vi "runTestScenario.vi"(8 "error in (no error)":errorcluster, 11 "Constant Analog Output Voltage Test  in":refnum<class "Modulated Analog Output Voltage Test.lvclass">) -> (0 "error out":errorcluster, 1 "Result":T1, 2 "TestExecution":T2, 3 "Constant Analog Output Voltage Test  out":refnum<class "Modulated Analog Output Voltage Test.lvclass">)   [LabVIEW 2015, in "Modulated Analog Output Voltage Test.lvclass"]
uses:
  Modulated Analog Output Voltage Test.lvclass
  Typedefs/TestExecution.ctl
  Typedefs/PassFailTest.ctl
  Modulated Analog Output Voltage Test.lvclass/Modulated Analog Output Voltage Test.ctl
  Typedefs/WriteDataFileInput.ctl
  Typedefs/TestScenarioTypes.ctl
  Typedefs/WriteLogMessageInput.ctl
  <vilib>/express/express arith-compare/Formula/XNode/ExpressFormulaBlockNode.xnode
  Model/TestLog/ITestLog/ITestLog.lvclass
  Model/ConverterStrategy/IConverterStrategy/IConverterStrategy.lvclass
  Model/ConfigureILCStrategy/IConfigureILCStrategy/IConfigureILCStrategy.lvclass
  Typedefs/ILCBTTypedefs.lvlib
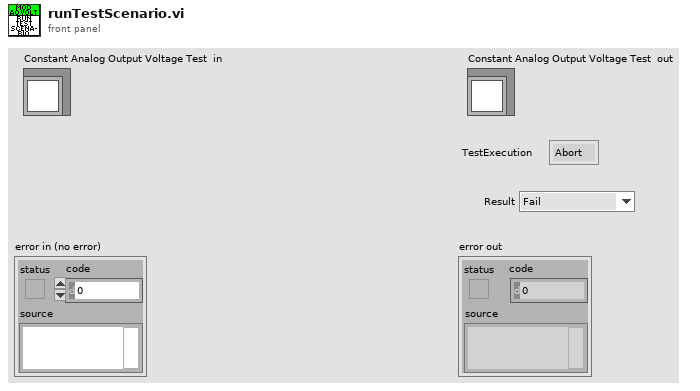
[diagram p1: front panel]
types:
  T1 = typedef "ILCBTTypedefs.lvlib/PassFailTest.ctl" = enum16{"Fail", "Pass", "NA"}
  T2 = typedef "ILCBTTypedefs.lvlib/TestExecution.ctl" = enum16{"Abort", "Continue"}
  T3 = typedef "ILCBTTypedefs.lvlib/WriteLogMessageInput.ctl" = cluster{"Test Scenario":T4, "Description":string, "Actual Value":string, "Data File":string, "Result":T1}
  T4 = typedef "ILCBTTypedefs.lvlib/TestScenarioTypes.ctl" = enum16{"+3.3VA Supply Test", "+3.3VD Supply Test", "+5VA Supply Test", "+5VD Supply Test", "Unique ID Test", "TEDS Status Test", "LIMSW1_TTL Low Test", "LIMSW1_TTL High Test", "LIMSW2_TTL Low Test", "LIMSW2_TTL High Test", "Tachometer Low Test", "Tachometer High Test", "SSR_TTL Low Test", "SSR_TTL High Test", "SM_GPI Low Test", "SM_GPI High Test", "CW Motion Without Limit Test", "CW Motion With Limit Test", "CW Motion With Both Limits Test", "CW Motion on CCW Limit Test", "CCW Motion Without Limit Test", "CCW Motion With Limit Test", "CCW Motion With Both Limits Test", "CCW Motion on CW Limit Test", "RS232-TXD Low Test", "RS232-TXD High Test", "RS232-RTS Low Test", "RS232-RTS High Test", "RS232-RXD Low Test", "RS232-RXD High Test", "RS232-CTS Low Test", "RS232-CTS High Test", "Out_SS Low Test", "Out_SS High Test", "Out_SDI Low Test", "Out_SDI High Test", "Out_SCLK Low Test", "Out_SCLK High Test", "Reset Low Test", "Reset High Test", "1 Channel ADC Test", "3 Channel ADC Test", "5 Channel ADC Test", "Vref Test", "ROT Test", "DAC1 Test", "DAC2 Test", "DAC3 Test", "DAC4 Test", "BIAS Test", "EXC1 Test", "EXC2 Test", "EXC3 Test", "EXC4 Test"}
  T5 = typedef "ILCBTTypedefs.lvlib/WriteDataFileInput.ctl" = cluster{"Test Scenario":T4, "File Name":string, "Output":string[]}
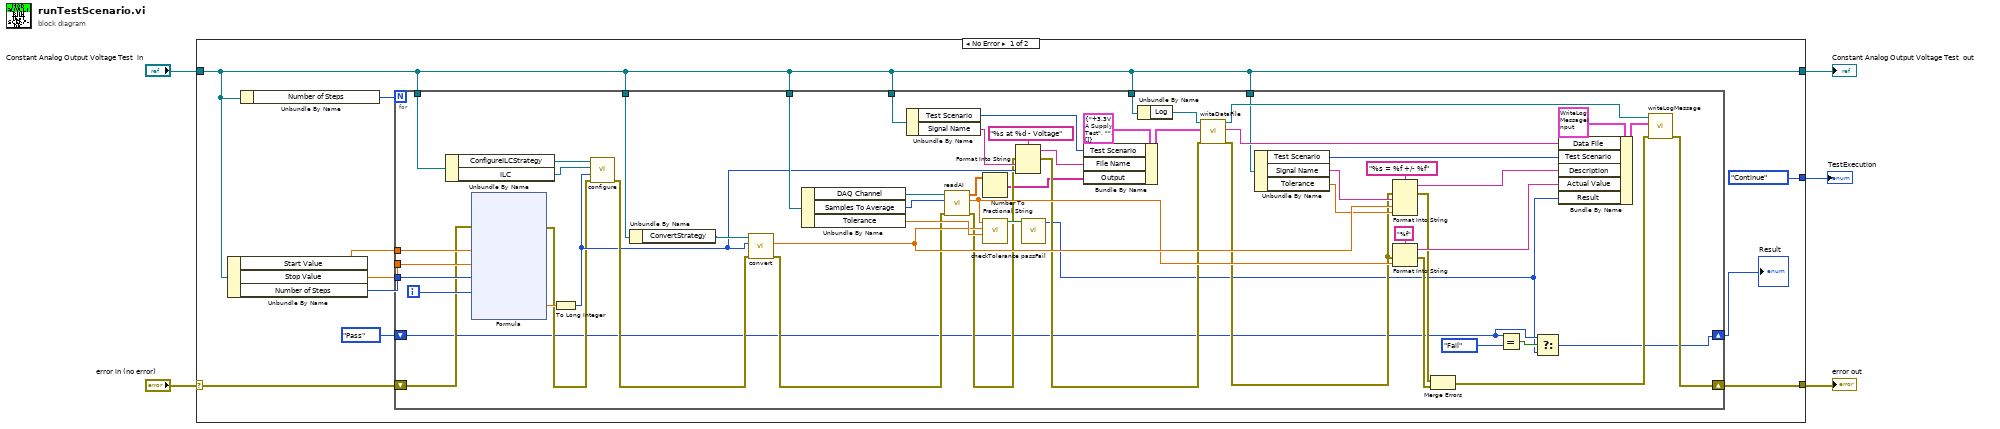
[diagram p0: block diagram]
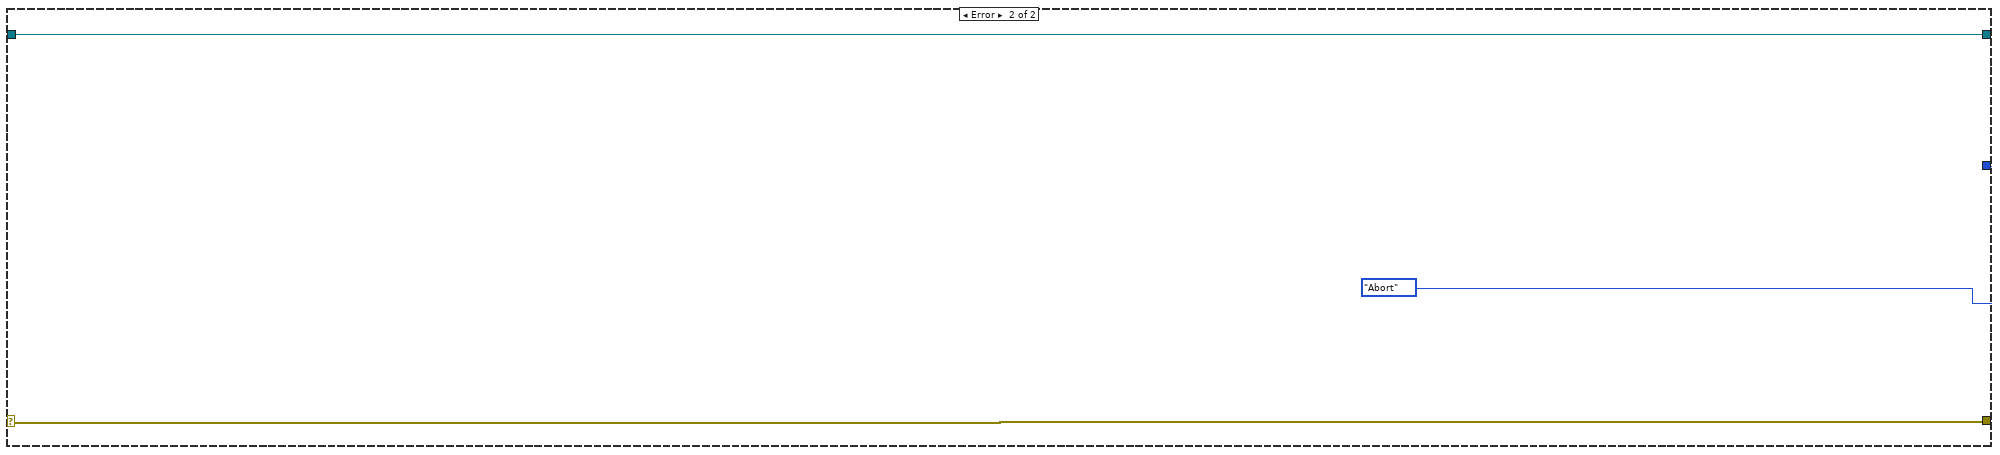
[diagram p2: hidden frame]
diagram:
  n1 = case shown="No Error" "error in (no error)" {
    selector: "error in (no error)" -> [w11 w89]
    tunnel: [w10 w89] -> w4
    tunnel: [TestExecution."Continue" ("TestExecution") TestExecution."Abort" ("TestExecution")] -> w3
    tunnel: "Constant Analog Output Voltage Test  in" -> [w8 w87]
    tunnel: [w8 w87] -> w1
    frame No Error {
      n2 = Unbundle By Name(w8) -> ("Start Value"=w14:dbl, "Stop Value"=w13:dbl, "Number of Steps"=w12:u16)
      n3 = Unbundle By Name(w8) -> ("Number of Steps"=w15:u16)
      n4 = for {
        N: w15 -> [_]
        tunnel: w8 -> [w70]
        tunnel: w14 -> [w69]
        tunnel: w13 -> [w68]
        tunnel: w12 -> [w67]
        tunnel: w8 -> [w64]
        tunnel: w8 -> [w60]
        tunnel: w8 -> [w55]
        tunnel: w8 -> [w52]
        shift-right: [w33] -> w10
        shift-left: w11 -> [w24]
        tunnel: w8 -> [w32]
        shift-right: [w16] -> w7
        shift-left: PassFailTest."Pass" ("Result") -> [w18]
        i -> [w66]
        n5 = Unbundle By Name(w70) -> ("ConfigureILCStrategy"=w71:refnum<class "IConfigureILCStrategy.lvclass">, "ILC"=w72:refnum<class "ILC.lvclass">)
        n6 = xnode "Formula"("START"=w69, "STOP"=w68, "NUM"=w67, "X"=w66, "error in (no error)"=w24) -> ("Result"=w65:dbl, "error out"=w23:errorcluster)
        n7 = To Long Integer(number=w65) -> (32bit integer=w29:i32)
        n8 = call-dynamic "configure.vi"("error in (no error)"=w23, "Value"=w29, "ILC"=w72, "IConfigureILCStrategy in"=w71) -> ("error out"=w35:errorcluster)  [unwired: 6 in, 1 out]
        n9 = Unbundle By Name(w64) -> ("ConvertStrategy"=w63:refnum<class "IConverterStrategy.lvclass">)
        n10 = call-dynamic "convert.vi"("error in (no error)"=w35, "Input"=w29, "IConverterStrategy in"=w63) -> ("error out"=w34:errorcluster, "Output"=w49:dbl)  [unwired: 6 in, 1 out]
        n11 = Unbundle By Name(w60) -> ("DAQ Channel"=w62:refnum<k21>, "Samples To Average"=w61:i32, "Tolerance"=w59:dbl)
        n12 = Unbundle By Name(w55) -> ("Test Scenario"=w57:T4, "Signal Name"=w30:string)
        n13 = call "readAI.vi"("error in (no error)"=w34, "Samples To Read"=w61, "DAQ Channel To Read"=w62) -> ("error out"=w28:errorcluster, "Average"=w47:dbl, "Samples"=w22:dbl[])  [unwired: 6 in]
        n14 = Number To Fractional String(number=w22) -> (F-format string=w21:string[])  [unwired: 3 in]
        n15 = call "checkTolerance.vi"("Tolerance"=w59, "Expected Value"=w49, "Average"=w47) -> ("Boolean"=w58:bool)  [unwired: 8 in]
        n16 = Format Into String(format string="%s at %d - Voltage", error in=w28, w30, w29) -> (resulting string=w31:string, error out=w27:errorcluster)  [unwired: 1 in]
        n17 = call "passFail.vi"("Boolean"=w58) -> ("Result"=w17:T1)  [unwired: 10 in]
        n18 = Bundle By Name(cluster=T5 {"Test Scenario"=enum."+3.3VA Supply Test", "File Name"="", "Output"=[]} ("WriteDataFileInput"), "Test Scenario"=w57, "File Name"=w31, "Output"=w21) -> (w54:T5)
        n19 = Unbundle By Name(w52) -> ("Log"=w53:refnum<class "ITestLog.lvclass">)
        n20 = call-dynamic "writeDataFile.vi"("error in (no error)"=w27, "WriteDataFileInput"=w54, "ITestLog in"=w53) -> ("error out"=w37:errorcluster, "Relative Path"=w41:string, "ITestLog out"=w40:refnum<class "ITestLog.lvclass">)  [unwired: 6 in]
        n21 = Unbundle By Name(w32) -> ("Test Scenario"=w42:T4, "Signal Name"=w50:string, "Tolerance"=w48:dbl)
        n22 = Format Into String(format string="%s = %f +/- %f", error in=w37, w50, w49, w48) -> (resulting string=w43:string, error out=w38:errorcluster)  [unwired: 1 in]
        n23 = Format Into String(format string="%f", error in=w37, w47) -> (resulting string=w44:string, error out=w39:errorcluster)  [unwired: 1 in]
        n24 = Merge Errors(w38, w39) -> (w36:errorcluster)
        n25 = Equal?(x=w18, y=PassFailTest."Fail") -> (x = y?=w19:bool)
        n26 = Select(t=w18, s=w19, f=w17) -> (s? t:f=w16:T1)
        n27 = Bundle By Name(cluster=T3 {"Test Scenario"=enum."+3.3VA Supply Test", "Description"="", "Actual Value"="", "Data File"="", "Result"=enum."Fail"} ("WriteLogMessageInput"), "Data File"=w41, "Test Scenario"=w42, "Description"=w43, "Actual Value"=w44, "Result"=w17) -> (w45:T3)
        n28 = call-dynamic "writeLogMessage.vi"("error in (no error)"=w36, "WriteLogMessageInput"=w45, "ITestLog in"=w40) -> ("error out"=w33:errorcluster)  [unwired: 7 in, 1 out]
      }
      "Result" <- w7
    }
    frame Error {
    }
  }
  "Constant Analog Output Voltage Test  out" <- w1
  "error out" <- w4
  "TestExecution" <- w3
